vi "Set_TriggerResponse.vi"(8 "error in":errorcluster, 10 "PicamTriggerResponse_":T1=1 items=["NoResponse"=1, "ReadoutPerTrigger"=2, "ShiftPerTrigger"=3, "ExposeDuringTriggerPulse"=4, "StartOnSingleTrigger"=5, "GatePerTrigger"=6], 11 "camera handle in":u64) -> (0 "error out":errorcluster, 3 "camera handle out":u64)   [LabVIEW 2019, in "PICam.lvlib"]
doc: "PicamAdcAnalogGain is the set of electronic gain settings for pixel digitization.\n\nPicamAdcAnalogGain_Low Small amplification.\nPicamAdcAnalogGain_Medium Average amplification.\nPicamAdcAnalogGain_High Large amplification.\n\nRefer to the user manual for the specific\ncamera being used for complete information."
uses:
  PICam.lvlib
  Ctrls/PicamTriggerResponse.ctl
  Picam64.dll   
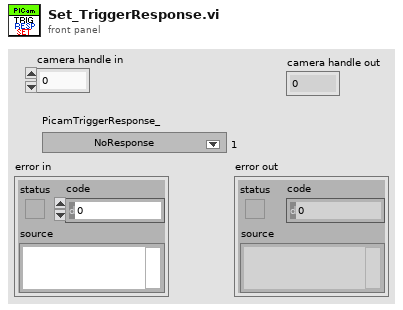
[diagram p1: front panel]
types:
  T1 = typedef "PICam.lvlib/PicamTriggerResponse.ctl" = u32
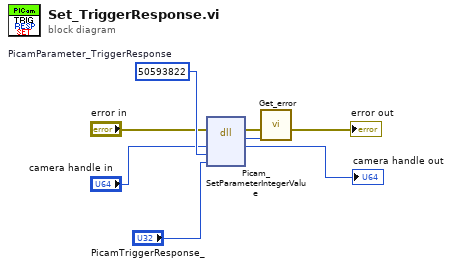
[diagram p0: block diagram]
diagram:
  w4 = u32 50593822  # PicamParameter_TriggerResponse
  n1 = dll-call lib="Picam32.dll" fn="Picam_SetParameterIntegerValue"(error in="error in", "camera"="camera handle in", "PicamParameter"=w4, "TriggerResponse"="PicamTriggerResponse_") -> (error out=w8:errorcluster, "return type"=w7:i32, "camera"=→"camera handle out":u64)  [unwired: 4 in, 1 out]
  n2 = call "Get_error.vi"("PICam_Error"=w7, "error in (no error)"=w8) -> ("error out"=→"error out":errorcluster)  [unwired: 9 in]
